vi "StagingBeamLine.vi"() -> ()   [LabVIEW 2020]
uses:
  SubVis/plungerstatus.ctl
  Controls/eventtypdef1.ctl
  Shared/GUI_Template/GUI_master/tcp new data cluster.ctl
panel:
  out "GUIdevice 13":string="StagingImageLocation"
  in  "DigitalOutput.Channel 0::12":bool caption="light"
  out "GUIdevice 12":string="StagingImageLocation"
  in  "JetStages>>JetStages":bool caption="JetStages"
  in  "laser trg":bool caption="Laser Trig."
  in  "Trigger Mode":bool caption="Laser Control"
  in  "Jet>>Jet2":bool caption="JetControl"
  out "ACave Diode Mirror>>XHair":u16(ring) caption="Diode Mirror"
  out "element":T1=enum."IN Beam"
  in  "Position.Channel 6::1":T2(ring) caption="Diode"
  in  "Filpper.Channel 7.Name::1":string="Beam2 Near" caption="Filpper.Channel 5.Name::1"
  in  "Filpper.Channel 6.Name::1":string="Beam2 Near" caption="Filpper.Channel 5.Name::1"
  in  "Position.Channel 7::1":T2(ring) caption="Beam 1 Dump"
  out "Boolean":bool
  in  "Fire button 2":bool caption="OK Button"
  in  "Fire button":bool caption="OK Button"
  in  "Spectrometer>>Spec":bool caption="Spectrometer"
  out "Diode\nFlipper":T3(ring)
  out "Energy\nFilter":T3(ring)
  in  "Uniblitz\nShutter":enum16{"Open", "Close", "Trigger", "Reset"}(ring)=enum."Close"
  out "Phosphor>>Plunger":u16(ring)
  in  "Dutch>>Magnet":bool caption="Mirror"
  out "Wedge>>Plunger":u16(ring)
  out "Beam Dump 2>>Plunger":u16(ring)
  out "Beam Dump 1>>Plunger":u16(ring)
  out "Beam2 Near_1>>XHair":u16(ring)
  out "Beam1 Far_1>>XHair":u16(ring)
  out "Beam1 Near_1>>XHair":u16(ring)
  out "Beam2 Far_2>>XHair":u16(ring)
  out "XH1_3>>XHair":u16(ring)
  in  "position.axis 2::11":dbl=3.999966 caption="OAPstage" min=0.0 max=50.0
  in  "position.axis 3::11":dbl=3.999966 caption="M5stage" min=0.0 max=50.0
  out "GUIdevice 11":string="StagingImageLocation"
  in  "position.channel 2::10":dbl=3.999966 caption="M4stage" min=0.0 max=25.0
  out "GUIdevice 10":string="StagingImageLocation"
  in  "position.channel 1::10":dbl=3.999966 caption="OAPstage" min=0.0 max=25.0
  in  "Position.Axis 5::9":dbl=-19.5 caption="CompPos" min=-49.0 max=51.0
  out "GUIdevice 9":string="StagingTRA3"
  in  "Position.Axis 1::8":dbl=36.99 caption="TelePos" min=0.0 max=150.0
  out "GUIdevice 8":string="StagingTelescopePosition"
  in  "Energy>>Energy":bool
  in  "StagingPhosphor>>Camera":bool caption="Phosphor"
  in  "StagingAlignBeam1>>Camera":bool caption="AlignBeam1"
  in  "StagingAlignBeam2>>Camera":bool caption="AlignBeam2"
  in  "time::7":dbl=-4.151986 caption="time (fs)" min=-2000000.0 max=2000000.0
  out "GUIdevice 7":string="StagingDelayStage"
  in  "position.Axis 1::13":dbl=34.3643 caption="DelayStagePos(mm)" min=0.0 max=54.0
  in  "DeviceControl":bool=TRUE
  in  "ignore interlock::6":bool=TRUE caption="ignore interlock"
  out "GUIdevice 6":string="StagingInterlock"
  out "fire interlock::6":bool caption="Interlock"
  in  "trigger.message::6":string
  in  "enableLaser::5":bool caption="Laser Trig."
  out "GUIdevice 5":string="StagingShotControl"
  out "fire::5":string
  in  "fire!!!":bool caption="fire"
  in  "Mode::5":bool caption="Laser Control"
  in  "position::4":dbl=-39.01 caption="ImagingPos" min=-75.0 max=50.0
  out "GUIdevice 4":string="StagingImageLocation"
  in  "position::3":dbl=10.000035 caption="FocusPos" min=-25.0 max=25.0
  in  "position::2":dbl=3.999966 caption="FocusPos" min=-100.0 max=100.0
  out "GUIdevice 3":string="StagingFocusPositionBeam2"
  out "GUIdevice 2":string="StagingFocusPositionBeam1"
  out "xnames":string[](array[string])=["XH1", "Beam2 Far", "Beam1 Near", "Beam1 Far", "Beam2 Near"]
  out "XHairs":refnum<vi>[](array[refnum])
  out "device status::1":string="no scan"
  in  "Filpper.Channel 5.Name::1":string="Beam2 Near"
  in  "Position.Channel 5::1":T2(ring)
  in  "Filpper.Channel 1.Name::1":string="XH1"
  in  "Filpper.Channel 2.Name::1":string="Beam2 Far"
  in  "Filpper.Channel 3.Name::1":string="Beam1 Near"
  in  "Filpper.Channel 4.Name::1":string="Beam1 Far"
  in  "Position.Channel 1::1":T2(ring)=enum."Unknown"
  in  "Position.Channel 2::1":T2(ring)
  in  "Position.Channel 3::1":T2(ring)
  in  "Position.Channel 4::1":T2(ring)
  out "GUIdevice 1":string="Staging1Wire"
  out "UDP error message":string
  in  "StagingOAP2Far>>Camera":bool caption="OAP2Far"
  in  "StagingOAP2Near>>Camera":bool caption="OAP2Near"
  in  "StagingM5>>Camera":bool caption="M5"
  in  "StagingM1Near>>Camera":bool caption="M1Near"
  in  "StagingM1Far>>Camera":bool caption="M1Far"
  in  "StagingM3Far>>Camera":bool caption="M3"
  in  "StagingM4>>Camera":bool caption="M4"
  in  "StagingOAP1Near>>Camera":bool caption="OAP1Near"
  in  "StagingOAP1Far>>Camera":bool caption="OAP1Far"
  in  "StagingModeTemp>>Camera":bool caption="Mode\nImager"
  in  "Caps>>Caps":bool caption="Caps"
  in  "hexapod>>hexapod":bool caption="hexapod"
  in  "OAP2>>Mirror":bool caption="Mirror"
  in  "DelayStageMotor 2":bool caption="OK Button"
  in  "DelayStageMotor 3":bool caption="OK Button"
  in  "M5>>Mirror":bool caption="Mirror"
  in  "StagingModeImager2>>Camera":bool caption="ModeImager2"
  in  "stop":bool
  in  "M4>>Mirror":bool caption="Mirror"
  in  "OAP1>>Mirror":bool caption="Mirror"
  in  "DelayStageMotor":bool caption="OK Button"
  in  "BS>>Mirror":bool caption="Mirror"
  in  "M1>>Mirror":bool caption="Mirror"
  in  "M3>>Mirror":bool caption="Mirror"
  out "Beam2":bool
  out "Tele":bool
  out "Beam1":bool
  out "after Phos":bool
  out "after Wedge":bool
  out "eBeam":bool
  out "fire":bool=TRUE
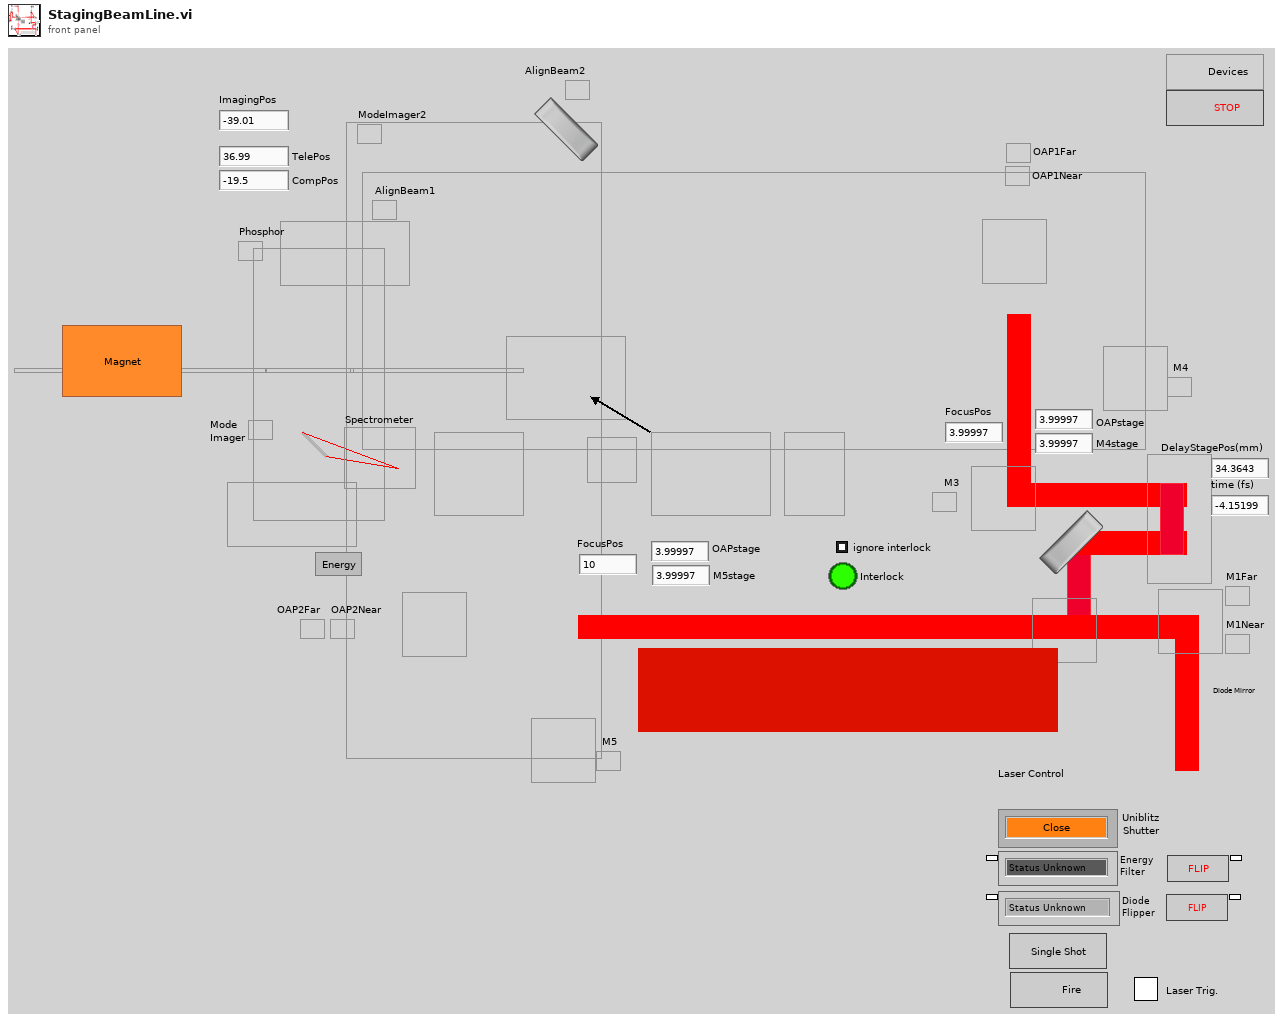
[diagram p1: front panel]
types:
  T1 = typedef "plungerstatus.ctl" = enum16{"unknown", "OUT of Beam", "IN Beam"}
  T2 = enum16{"Removed", "Inserted", "Unknown", "Moving"}
  T3 = enum16{"Status Unknown", "Flipper IN", "Flipper OUT"}
  T4 = enum16{"Read", "Write", "ReadWrite", "BufferedRead", "BufferedReadWrite"}
  T5 = typedef "tcp new data cluster.ctl" = cluster{"EventEnum":enum16{"new data", "connection status update"}, "Device name":string}
  T6 = typedef "eventtypdef1.ctl" = cluster{"label":string, "Sub Panel":refnum<vi>, "CtlRef":refnum<vi>, "This VI":refnum<vi>}
  T7 = enum8{"Enabled", "Disabled", "Disabled and Grayed Out"}
  T8 = enum16{"Beam Dump 1", "Beam Dump 2", "Wedge", "Phosphor"}
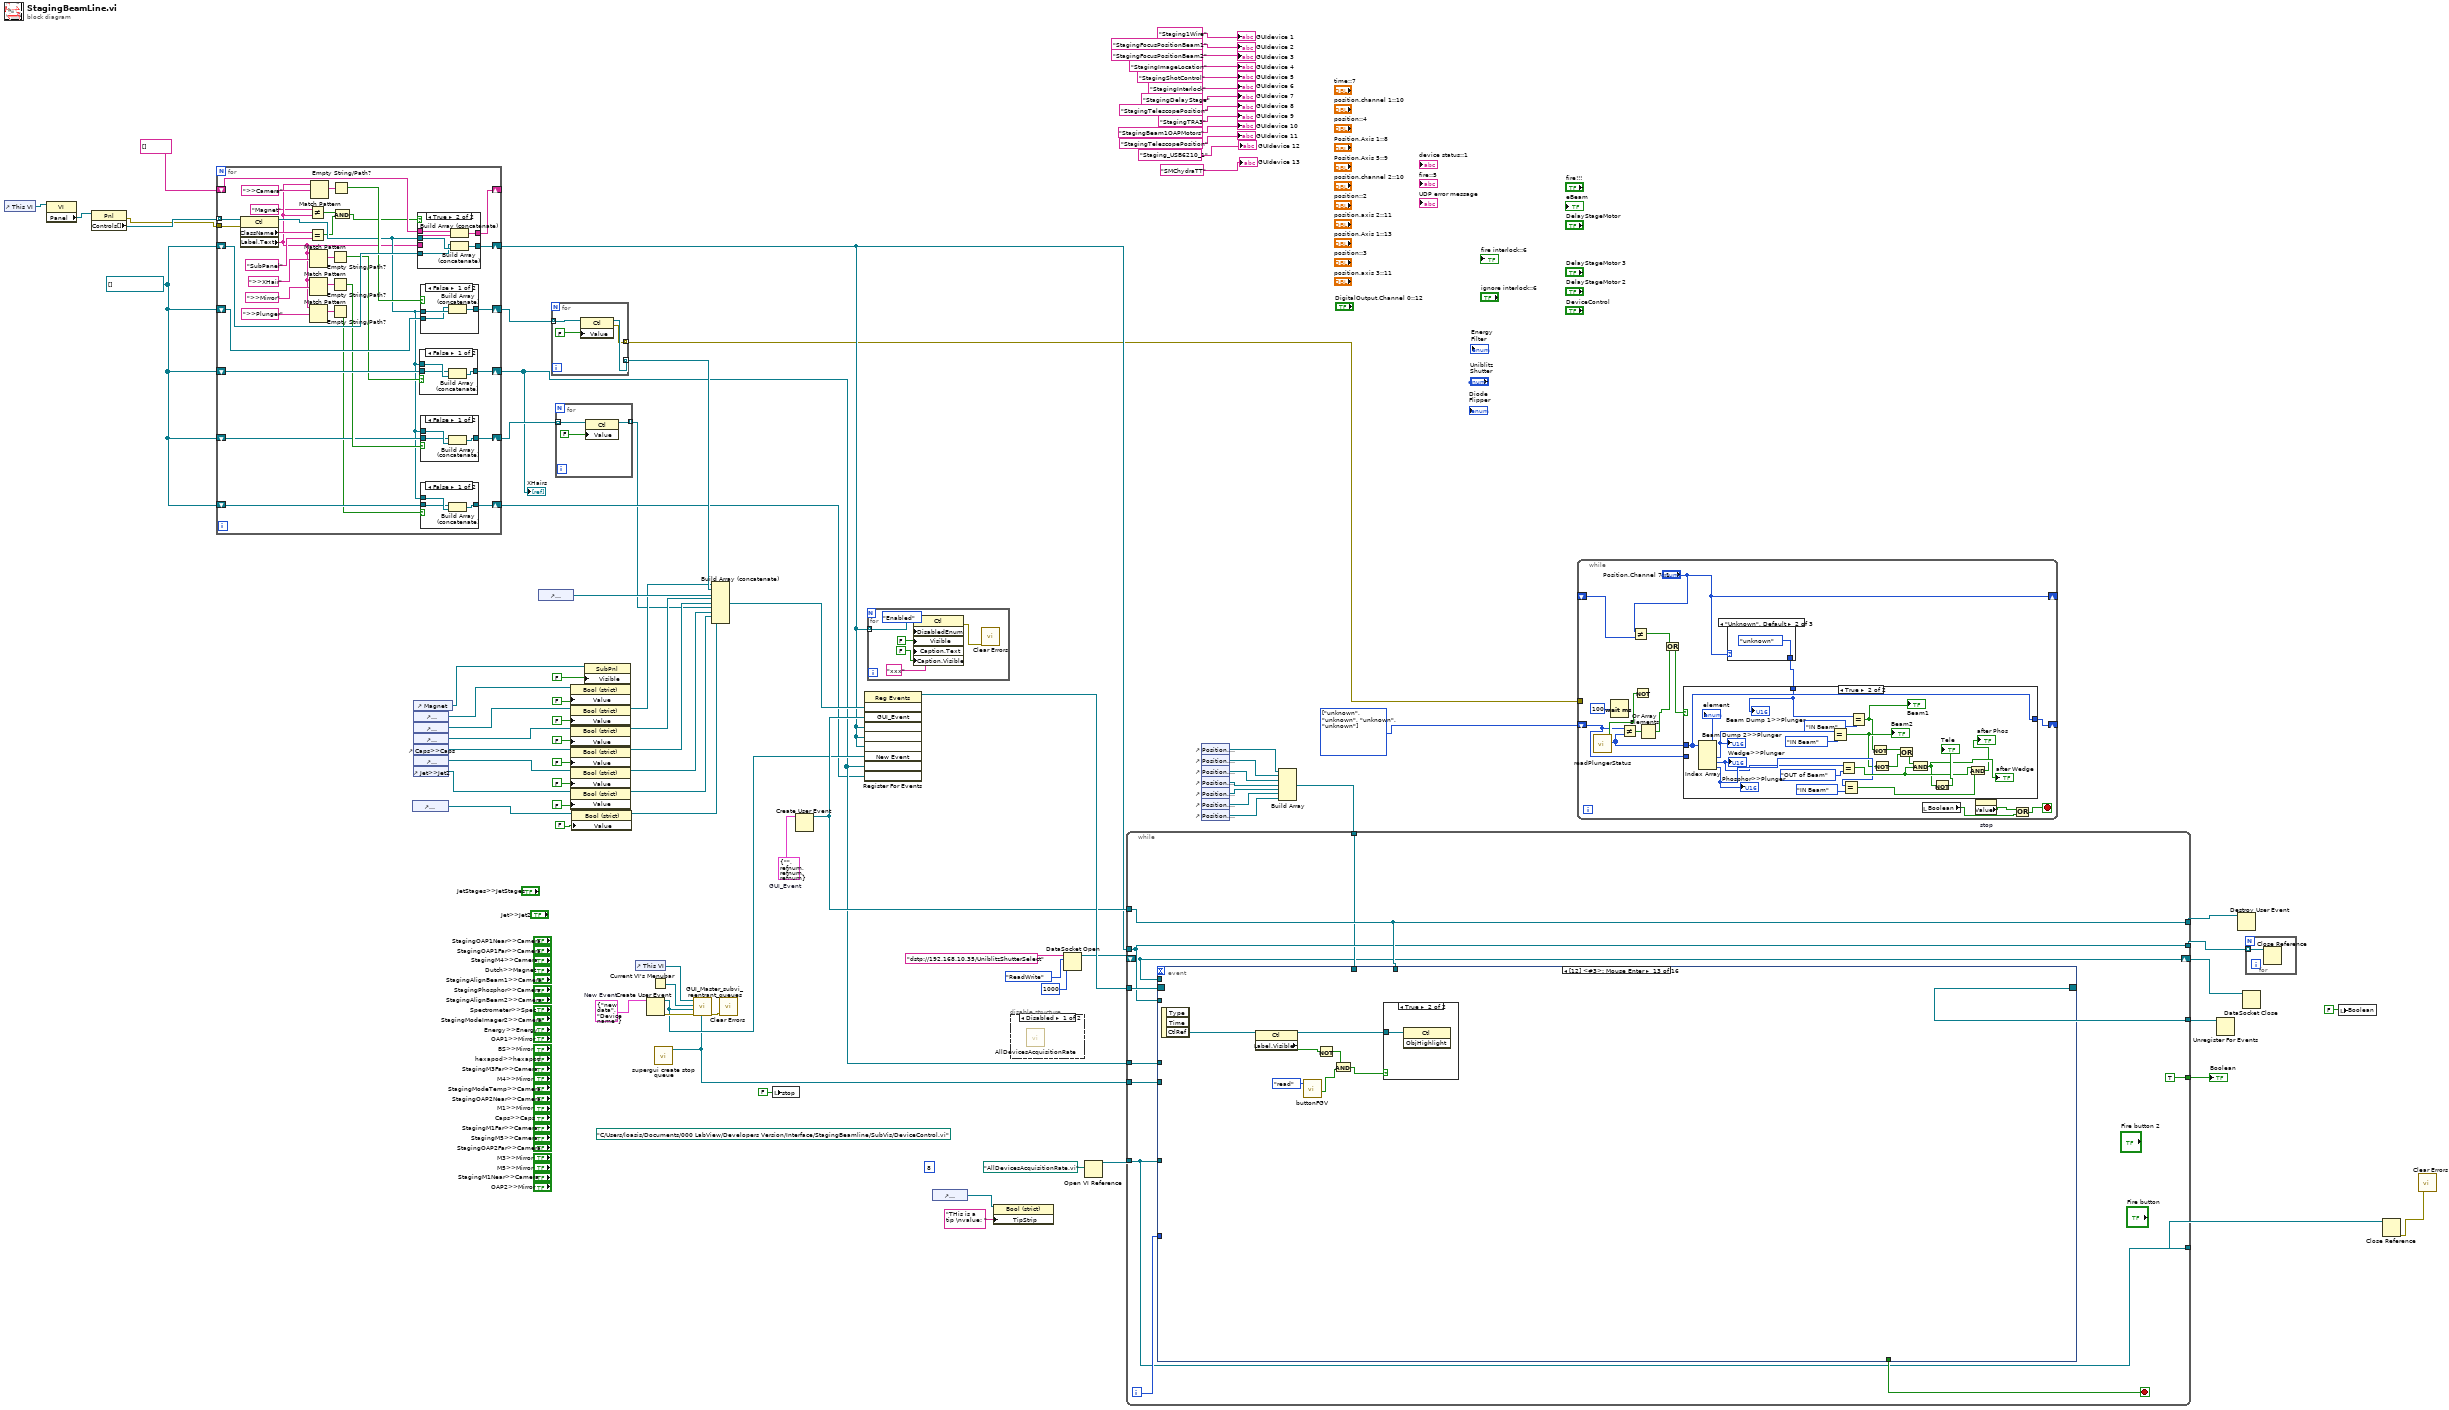
[diagram p0: block diagram]
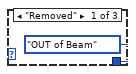
[diagram p2: hidden frame]
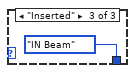
[diagram p3: hidden frame]
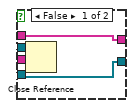
[diagram p10: hidden frame]
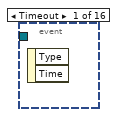
[diagram p11: hidden frame]
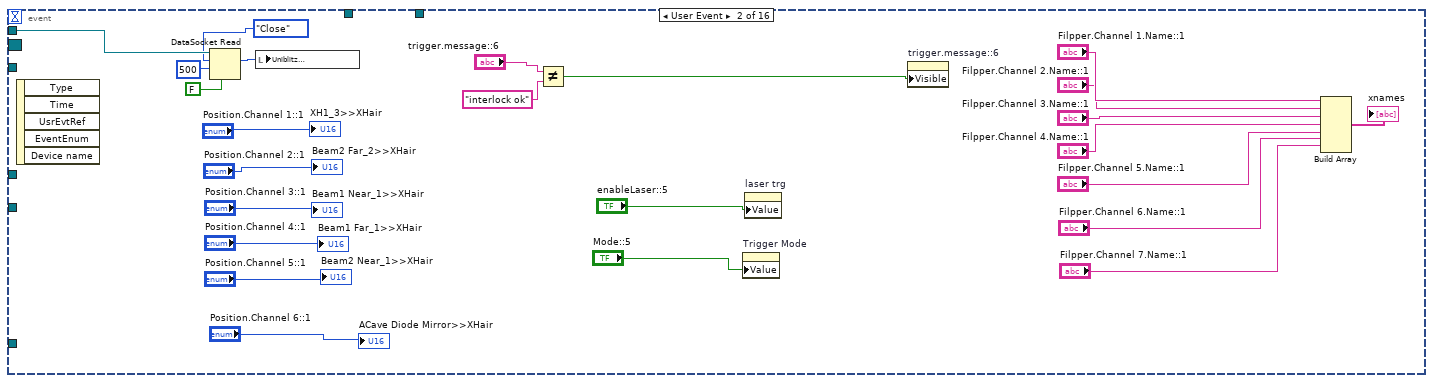
[diagram p12: hidden frame]
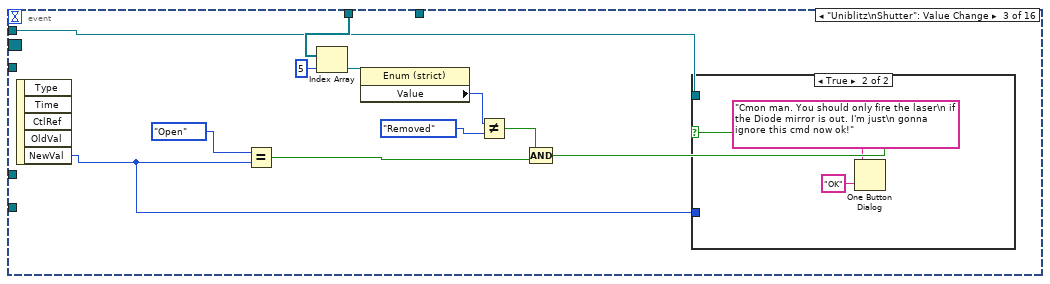
[diagram p13: hidden frame]
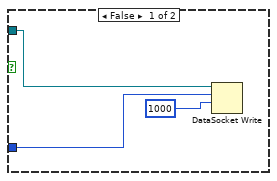
[diagram p14: hidden frame]
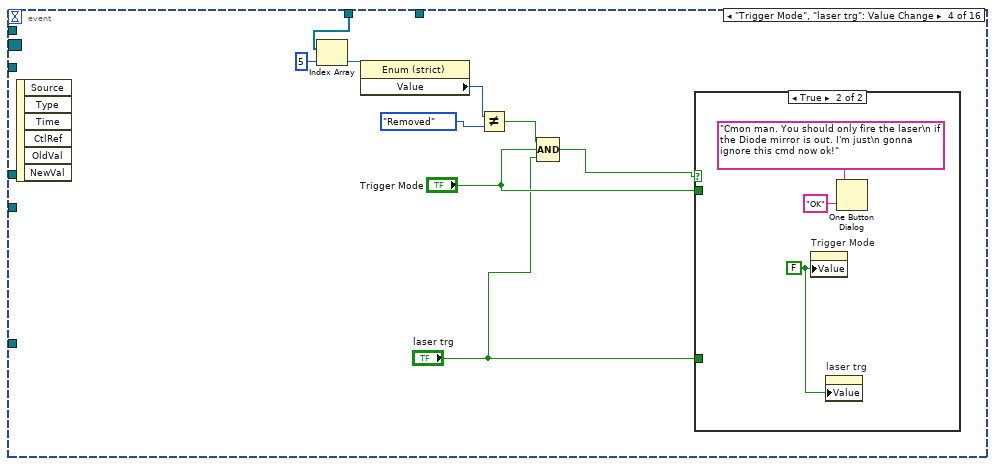
[diagram p15: hidden frame]
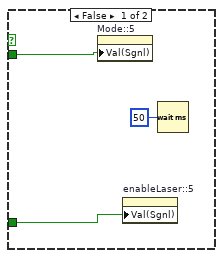
[diagram p16: hidden frame]
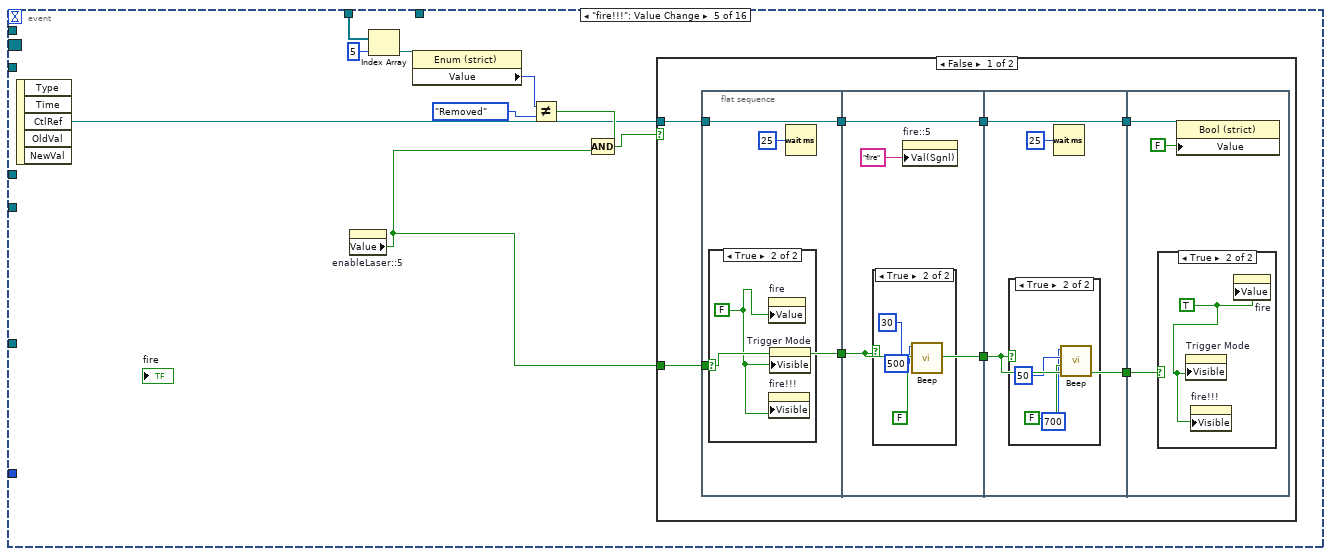
[diagram p17: hidden frame]
diagram:
  w31 = T1[] [enum."unknown", enum."unknown", enum."unknown", enum."unknown"] items=["unknown", "OUT of Beam", "IN Beam"] ("read switches")
  (unwired) path "C:/Users/loasis/Documents/000 LabView/Developers Version/Interface/StagingBeamline/SubVis/DeviceControl.vi" ("Path")
  (unwired) 8 ("options")
  w72 = T5 {"EventEnum"=enum."new data", "Device name"="Device name"}  # New Event
  w40 = refnum<vi>[] []
  w86 = T6 {"label"="", "Sub Panel"=refnum, "CtlRef"=refnum, "This VI"=refnum}  # GUI_Event
  n1 = control-ref of="This VI"() -> (w82:refnum<vi>)
  n2 = property class="VI"(reference=w82) -> ("Panel"=w81:refnum<vi>)  [unwired: 1 in, 2 out]
  n3 = property class="Pnl"(reference=w81) -> (error out=w79:errorcluster, "Controls[]"=w80:refnum<vi>[])  [unwired: 1 in, 1 out]
  n4 = for {
    tunnel: w80 -> [w120] mode=indexing
    tunnel: w79 -> [w121]
    shift-right: [w117] -> _
    shift-left: string[] [] -> [w116]
    shift-right: [w115] -> w75
    shift-left: w40 -> [w114]
    shift-right: [w110] -> w63
    shift-left: w40 -> [w109]
    shift-right: [w108] -> w42
    shift-left: w40 -> [w107]
    shift-right: [w100] -> w53
    shift-left: w40 -> [w99]
    shift-right: [w96] -> w39
    shift-left: w40 -> [w97]
    n5 = property class="Ctl"(reference=w120, error in=w121) -> (reference out=w98:refnum<vi>, "ClassName"=w119:string, "Label.Text"=w92:string)  [unwired: 1 out]
    n6 = Not Equal?(x="Magnet", y=w92) -> (x != y?=w90:bool)
    n7 = Equal?(x=w119, y="SubPanel") -> (x = y?=w88:bool)
    n8 = Match Pattern(string=w92, regular expression=">>XHair") -> (match substring=w105:string)  [unwired: 1 in, 3 out]
    n9 = Match Pattern(string=w92, regular expression=">>Mirror") -> (match substring=w102:string)  [unwired: 1 in, 3 out]
    n10 = Match Pattern(string=w92, regular expression=">>Plunger") -> (match substring=w94:string)  [unwired: 1 in, 3 out]
    n11 = Match Pattern(string=w92, regular expression=">>Camera") -> (match substring=w112:string)  [unwired: 1 in, 3 out]
    n12 = Empty String/Path?(string/path=w105) -> (empty?=w104:bool)
    n13 = Empty String/Path?(string/path=w102) -> (empty?=w103:bool)
    n14 = Empty String/Path?(string/path=w94) -> (empty?=w93:bool)
    n15 = Empty String/Path?(string/path=w112) -> (empty?=w111:bool)
    n16 = And(x=w90, y=w88) -> (x .and. y?=w89:bool)
    n17 = case shown="True" w89 {
      tunnel: w98 -> [w140 w143]
      tunnel: w92 -> [_ w146]
      tunnel: [w139 w145] -> w117
      tunnel: w116 -> [w139 w144]
      tunnel: [w138 w142] -> w115
      tunnel: w114 -> [w138 w141]
      frame False {
        n18 = Close Reference(reference=w140) -> ()  [unwired: 1 in, 1 out]
      }
      frame True {
        n19 = Build Array (concatenate)(w144, w146) -> (w145:string[])
        n20 = Build Array (concatenate)(w141, w143) -> (w142:refnum<vi>[])
      }
    }
    n21 = case shown="False" w104 {
      tunnel: w98 -> [w132 _]
      tunnel: [w131 w133] -> w108
      tunnel: w107 -> [w130 w133]
      frame False {
        n22 = Build Array (concatenate)(w130, w132) -> (w131:refnum<vi>[])
      }
      frame True {
      }
    }
    n23 = case shown="False" w111 {
      tunnel: w98 -> [w136 _]
      tunnel: [w135 w137] -> w110
      tunnel: w109 -> [w134 w137]
      frame False {
        n24 = Build Array (concatenate)(w134, w136) -> (w135:refnum<vi>[])
      }
      frame True {
      }
    }
    n25 = case shown="False" w103 {
      tunnel: w98 -> [w128 _]
      tunnel: [w127 w129] -> w100
      tunnel: w99 -> [w126 w129]
      frame False {
        n26 = Build Array (concatenate)(w126, w128) -> (w127:refnum<vi>[])
      }
      frame True {
      }
    }
    n27 = case shown="False" w93 {
      tunnel: w98 -> [w124 _]
      tunnel: [w123 w125] -> w96
      tunnel: w97 -> [w122 w125]
      frame False {
        n28 = Build Array (concatenate)(w122, w124) -> (w123:refnum<vi>[])
      }
      frame True {
      }
    }
  }
  "XHairs" <- w42
  n29 = control-ref of="JetStages>>JetStages"() -> (w5:refnum<vi>)
  n30 = control-ref of="Magnet"() -> (w35:refnum<vi>)
  n31 = control-ref of="Dutch>>Magnet"() -> (w38:refnum<vi>)
  n32 = control-ref of="Energy>>Energy"() -> (w49:refnum<vi>)
  n33 = control-ref of="hexapod>>hexapod"() -> (w59:refnum<vi>)
  n34 = control-ref of="Caps>>Caps"() -> (w61:refnum<vi>)
  n35 = control-ref of="Spectrometer>>Spec"() -> (w34:refnum<vi>)
  n36 = control-ref of="Jet>>Jet2"() -> (w16:refnum<vi>)
  n37 = control-ref of="StagingModeImager2>>Camera"() -> (w85:refnum<vi>)
  n38 = for {
    tunnel: w63 -> [w150] mode=indexing
    tunnel: [w148] -> w62 mode=indexing
    tunnel: [w147] -> w27 mode=indexing
    n39 = property class="Ctl"(reference=w150, "Value"=FALSE ("Visible")) -> (reference out=w148:refnum<vi>, error out=w147:errorcluster)  [unwired: 1 in]
  }
  n40 = for {
    tunnel: w53 -> [w153] mode=indexing
    tunnel: [w151] -> w14 mode=indexing
    n41 = property class="Ctl"(reference=w153, "Value"=FALSE ("Visible")) -> (reference out=w151:refnum<vi>)  [unwired: 1 in, 1 out]
  }
  n42 = property class="Bool (strict)"(reference=w38, "Value"=FALSE) -> ()  [unwired: 1 in, 2 out]
  n43 = property class="Bool (strict)"(reference=w49, "Value"=FALSE) -> (reference out=w47:refnum<vi>)  [unwired: 1 in, 1 out]
  n44 = property class="Bool (strict)"(reference=w59, "Value"=FALSE) -> (reference out=w58:refnum<vi>)  [unwired: 1 in, 1 out]
  n45 = property class="Bool (strict)"(reference=w61, "Value"=FALSE) -> (reference out=w19:refnum<vi>)  [unwired: 1 in, 1 out]
  n46 = property class="Bool (strict)"(reference=w34, "Value"=FALSE) -> (reference out=w32:refnum<vi>)  [unwired: 1 in, 1 out]
  n47 = property class="Bool (strict)"(reference=w16, "Value"=FALSE) -> (reference out=w15:refnum<vi>)  [unwired: 1 in, 1 out]
  n48 = property class="Bool (strict)"(reference=w5, "Value"=FALSE) -> (reference out=w4:refnum<vi>)  [unwired: 1 in, 1 out]
  n49 = property class="SubPnl"(reference=w35, "Visible"=FALSE) -> ()  [unwired: 1 in, 2 out]
  n50 = control-ref of="This VI"() -> (w70:refnum<vi>)
  n51 = Create User Event(user event datatype=w72) -> (user event=w69:refnum<user-event>, error out=w73:errorcluster)  [unwired: 1 in]
  n52 = Current VI's Menubar() -> (w71:refnum<k9>)
  n53 = call "supergui create stop queue.vi"() -> ("STOP Queue out"=w1:refnum<queue>)  [unwired: 11 in]
  n54 = call "GUI_Master_subvi_reentrant_queues.vi"("STOP Queue in"=w1, "error in (no error)"=w73, "tcp data event"=w69, "Caller menu reference"=w71, "Caller VI ref"=w70) -> ("error out"=w74:errorcluster)  [unwired: 6 in]
  n55 = Build Array (concatenate)(w47, w62, w85, w58, w19, w14, w32, w15, w4) -> (w84:refnum<vi>[])
  n56 = call <vilib>:"Clear Errors.vi"("error in (no error)"=w74) -> ()  [unwired: 5 in, 2 out]
  n57 = local write "stop"(FALSE ("stop")) -> ()
  n58 = Create User Event(user event datatype=w86) -> (user event=w76:refnum<user-event>)  [unwired: 1 in, 1 out]
  n59 = register-events(w84, w76, w75, w75, w75, w69, w42, w39) -> (reference out=w83:refnum<event-registration>)  [unwired: 2 in, 1 out]
  n60 = for {
    tunnel: w75 -> [w158] mode=indexing
    n61 = property class="Ctl"(reference=w158, "DisabledEnum"=T7."Enabled" ("Disabled"), "Visible"=FALSE, "Caption.Text"="xxx", "Caption.Visible"=FALSE ("Label.Visible")) -> (error out=w154:errorcluster)  [unwired: 1 in, 1 out]
    n62 = call <vilib>:"Clear Errors.vi"("error in (no error)"=w154) -> ()  [unwired: 5 in, 2 out]
  }
  n63 = control-ref of="DelayStageMotor"() -> (w44:refnum<vi>)
  n64 = property class="Bool (strict)"(reference=w44, "TipStrip"="THis is a tip \nvalue: ") -> ()  [unwired: 1 in, 2 out]
  n65 = disable-structure shown="Disabled" {
    frame Disabled {
      n66 = call "AllDevicesAcquisitionRate.vi"() -> ()  [unwired: 11 in, 1 out]
    }
    frame Enabled {
    }
  }
  n67 = DataSocket Open(9:1000 ("ms timeout (10000)"), 10:T4."ReadWrite" ("mode"), 11:"dstp://192.168.10.35/UniblitzShutterSelect" ("URL")) -> (3:w26:refnum<k13>)  [unwired: 1 in, 1 out]
  n68 = Open VI Reference(vi path=path "AllDevicesAcquisitionRate.vi" ("Path")) -> (vi reference=w54:refnum<vi>)  [unwired: 5 in, 1 out]
  n69 = control-ref of="Position.Channel 1::1"() -> (w64:refnum<vi>)
  n70 = control-ref of="Position.Channel 2::1"() -> (w65:refnum<vi>)
  n71 = control-ref of="Position.Channel 3::1"() -> (w66:refnum<vi>)
  n72 = control-ref of="Position.Channel 4::1"() -> (w67:refnum<vi>)
  n73 = control-ref of="Position.Channel 5::1"() -> (w68:refnum<vi>)
  n74 = control-ref of="Position.Channel 6::1"() -> (w21:refnum<vi>)
  n75 = control-ref of="Position.Channel 7::1"() -> (w20:refnum<vi>)
  n76 = Build Array(w64, w65, w66, w67, w68, w21, w20) -> (w18:refnum<vi>[])
  n77 = while {
    tunnel: w76 -> [w170]
    tunnel: [w170] -> w87
    tunnel: w83 -> [w169]
    tunnel: w75 -> [w168]
    tunnel: [w168] -> w77
    tunnel: w42 -> [w166]
    tunnel: w18 -> [w165]
    tunnel: [w164] -> w56
    tunnel: w54 -> [w164]
    tunnel: [w163] -> w41
    tunnel: [TRUE] -> w29
    shift-right: [w161] -> w25
    shift-left: w26 -> [w161]
    tunnel: w1 -> [w160]
    i -> [w167]
    stop <- w171 stop-if-true
    n78 = event shown="[12] <#3>: Mouse Enter" {
      selector: w169 -> [_ _ _ _ _ _ _ _ _ _ _ _ _ _ _ _]
      dyn-events: [_ _ _ _ _ _ _ _ _ _ _ _ _ _ _ _] -> w163
      timeout: _ -> [_ _ _ _ _ _ _ _ _ _ _ _ _ _ _ _]
      tunnel: [_ _ _ _ _ _ _ _ _ _ _ _ _ _ _ "stop"] -> w171
      tunnel: w170 -> [_ _ _ _ _ _ _ _ w305 w309 _ _ _ _ _ w395]
      tunnel: w168 -> [_ _ _ _ _ _ _ _ w304 w307 _ w334 _ _ _ _]
      tunnel: w167 -> [_ _ _ _ _ _ _ _ _ _ _ _ _ _ _ _]
      tunnel: w166 -> [_ _ _ _ _ _ _ _ _ _ _ _ _ _ _ _]
      tunnel: w165 -> [_ _ w206 w216 w231 w276 _ _ _ _ _ _ _ _ _ _]
      tunnel: w164 -> [_ _ _ _ _ _ _ _ _ _ w317 _ _ _ _ _]
      tunnel: w161 -> [_ w181 w196 _ _ _ _ _ _ _ _ _ _ _ _ _]
      tunnel: w160 -> [_ _ _ _ _ _ _ _ _ _ _ _ _ _ _ w388]
      event Timeout {
        n79 = event-data() -> ()  [unwired: 1 in, 2 out]
      }
      event User Event {
        n80 = event-data() -> ()  [unwired: 1 in, 5 out]
        n81 = DataSocket Read(6:FALSE ("wait for updated value (T)"), 9:500 ("ms timeout (10000)"), 10:enum16{"Open", "Close", "Trigger", "Reset"}."Close" ("Uniblitz\nShutter 2"), 11:w181) -> (2:w179:enum16{"Open", "Close", "Trigger", "Reset"})  [unwired: 1 in, 6 out]
        n82 = local write "Uniblitz\nShutter"(w179) -> ()
        n83 = Not Equal?(x="trigger.message::6", y="interlock ok") -> (x != y?=w182:bool)
        n84 = property on="Trigger Mode" class="Bool (strict)"("Value"="Mode::5") -> ()  [unwired: 2 in, 2 out]
        n85 = property on="laser trg" class="Bool (strict)"("Value"="enableLaser::5") -> ()  [unwired: 2 in, 2 out]
        n86 = property on="trigger.message::6" class="Str"("Visible"=w182) -> ()  [unwired: 2 in, 2 out]
        n87 = Build Array("Filpper.Channel 1.Name::1", "Filpper.Channel 2.Name::1", "Filpper.Channel 3.Name::1", "Filpper.Channel 4.Name::1", "Filpper.Channel 5.Name::1", "Filpper.Channel 6.Name::1", "Filpper.Channel 7.Name::1") -> (→"xnames":string[])
        "XH1_3>>XHair" <- "Position.Channel 1::1"
        "Beam2 Far_2>>XHair" <- "Position.Channel 2::1"
        "Beam1 Near_1>>XHair" <- "Position.Channel 3::1"
        "Beam1 Far_1>>XHair" <- "Position.Channel 4::1"
        "Beam2 Near_1>>XHair" <- "Position.Channel 5::1"
        "ACave Diode Mirror>>XHair" <- "Position.Channel 6::1"
      }
      event "Uniblitz\nShutter": Value Change {
        n88 = event-data() -> ("NewVal"=w197:enum16{"Open", "Close", "Trigger", "Reset"})  [unwired: 1 in, 4 out]
        n89 = Equal?(x=enum16{"Open", "Close", "Trigger", "Reset"}."Open" ("Uniblitz\nShutter"), y=w197) -> (x = y?=w199:bool)
        n90 = Index Array(array=w206, index=5) -> (element=w204:refnum<vi>)
        n91 = property class="Enum (strict)"(reference=w204) -> ("Value"=w201:T2)  [unwired: 1 in, 2 out]
        n92 = Not Equal?(x=w201, y=T2."Removed" ("Position.Channel 6::1")) -> (x != y?=w200:bool)
        n93 = Compound Arithmetic op=AND(w200, w199) -> (w198:bool)
        n94 = case shown="True" w198 {
          tunnel: w197 -> [w208 _]
          tunnel: w196 -> [w207 _]
          frame False {
            n95 = DataSocket Write(9:1000 ("ms timeout (0)"), 10:w208, 11:w207) -> ()  [unwired: 1 in, 3 out]
          }
          frame True {
            n96 = One Button Dialog(message="Cmon man. You should only fire the laser\n if the Diode mirror is out. I'm just\n gonna ignore this cmd now ok!", button name ("OK")="OK") -> ()  [unwired: 1 out]
          }
        }
      }
      event "Trigger Mode", "laser trg": Value Change {
        n97 = event-data() -> ()  [unwired: 1 in, 6 out]
        n98 = Index Array(array=w216, index=5) -> (element=w219:refnum<vi>)
        n99 = property class="Enum (strict)"(reference=w219) -> ("Value"=w217:T2)  [unwired: 1 in, 2 out]
        n100 = Not Equal?(x=w217, y=T2."Removed" ("Position.Channel 6::1")) -> (x != y?=w215:bool)
        n101 = Compound Arithmetic op=AND(w215, "Trigger Mode", "laser trg") -> (w214:bool)
        n102 = case shown="True" w214 {
          tunnel: "Trigger Mode" -> [w223 _]
          tunnel: "laser trg" -> [w222 _]
          frame False {
            n103 = property on="Mode::5" class="Bool (strict)"("Val(Sgnl)"=w223) -> ()  [unwired: 2 in, 2 out]
            n104 = property on="enableLaser::5" class="Bool (strict)"("Val(Sgnl)"=w222) -> ()  [unwired: 2 in, 2 out]
            n105 = Wait (ms)(milliseconds to wait=u32 50) -> ()  [unwired: 1 out]
          }
          frame True {
            w224 = FALSE ("Trigger Mode")
            n106 = property on="Trigger Mode" class="Bool (strict)"("Value"=w224) -> ()  [unwired: 2 in, 2 out]
            n107 = property on="laser trg" class="Bool (strict)"("Value"=w224) -> ()  [unwired: 2 in, 2 out]
            n108 = One Button Dialog(message="Cmon man. You should only fire the laser\n if the Diode mirror is out. I'm just\n gonna ignore this cmd now ok!", button name ("OK")="OK") -> ()  [unwired: 1 out]
          }
        }
      }
      event "fire!!!": Value Change {
        n109 = event-data() -> ("CtlRef"=w228:refnum<vi>)  [unwired: 1 in, 4 out]
        n110 = property on="enableLaser::5" class="Bool (strict)"() -> ("Value"=w227:bool)  [unwired: 2 in, 2 out]
        n111 = Index Array(array=w231, index=5) -> (element=w234:refnum<vi>)
        n112 = property class="Enum (strict)"(reference=w234) -> ("Value"=w232:T2)  [unwired: 1 in, 2 out]
        n113 = Not Equal?(x=w232, y=T2."Removed" ("Position.Channel 6::1")) -> (x != y?=w230:bool)
        n114 = Compound Arithmetic op=AND(w230, w227) -> (w229:bool)
        n115 = case shown="False" w229 {
          tunnel: w228 -> [w240 w264]
          tunnel: w227 -> [w239 _]
          frame False {
            n116 = flat-sequence {
              tunnel: [w245] -> w241
              tunnel: w240 -> [w245]
              tunnel: w239 -> [w244]
              tunnel: [w244] -> w238
              tunnel: [w249] -> w242
              tunnel: w241 -> [w249]
              tunnel: w238 -> [w248]
              tunnel: [w248] -> w237
              tunnel: [w255] -> w243
              tunnel: w242 -> [w255]
              tunnel: w237 -> [w254]
              tunnel: [w254] -> w236
              tunnel: w243 -> [w261]
              tunnel: w236 -> [w260]
              frame #0 {
                n117 = case shown="True" w244 {
                  frame False {
                  }
                  frame True {
                    w247 = FALSE ("fire ind")
                    n118 = property on="fire" class="Bool (strict)"("Value"=w247) -> ()  [unwired: 2 in, 2 out]
                    n119 = property on="fire!!!" class="Bool (strict)"("Visible"=w247) -> ()  [unwired: 2 in, 2 out]
                    n120 = property on="Trigger Mode" class="Bool (strict)"("Visible"=w247) -> ()  [unwired: 2 in, 2 out]
                  }
                }
                n121 = Wait (ms)(milliseconds to wait=u32 25) -> ()  [unwired: 1 out]
              }
              frame #1 {
                n122 = case shown="True" w248 {
                  frame False {
                  }
                  frame True {
                    n123 = call <vilib>:"Beep.vi"("use system alert? (T)"=FALSE ("use system alert? (T) 2"), "duration (msec)"=u32 30 ("duration (msec) 2"), "frequency (Hz)"=u32 500 ("frequency (Hz) 2")) -> ()  [unwired: 9 in]
                  }
                }
                n124 = property on="fire::5" class="Str"("Val(Sgnl)"="fire" ("fire::5")) -> ()  [unwired: 2 in, 2 out]
              }
              frame #2 {
                n125 = case shown="True" w254 {
                  frame False {
                  }
                  frame True {
                    n126 = call <vilib>:"Beep.vi"("use system alert? (T)"=FALSE, "duration (msec)"=u32 50, "frequency (Hz)"=u32 700) -> ()  [unwired: 9 in]
                  }
                }
                n127 = Wait (ms)(milliseconds to wait=u32 25) -> ()  [unwired: 1 out]
              }
              frame #3 {
                n128 = case shown="True" w260 {
                  frame False {
                  }
                  frame True {
                    w263 = TRUE ("fire ind")
                    n129 = property on="Trigger Mode" class="Bool (strict)"("Visible"=w263) -> ()  [unwired: 2 in, 2 out]
                    n130 = property on="fire!!!" class="Bool (strict)"("Visible"=w263) -> ()  [unwired: 2 in, 2 out]
                    n131 = property on="fire" class="Bool (strict)"("Value"=w263) -> ()  [unwired: 2 in, 2 out]
                  }
                }
                n132 = property class="Bool (strict)"(reference=w261, "Value"=FALSE) -> ()  [unwired: 1 in, 2 out]
              }
            }
          }
          frame True {
            n133 = One Button Dialog(message="Cmon man. You should only fire the laser\n if the Diode mirror is out. I'm just\n gonna ignore this cmd now ok!", button name ("OK")="OK") -> ()  [unwired: 1 out]
            n134 = property class="Bool (strict)"(reference=w264, "Value"=FALSE) -> ()  [unwired: 1 in, 2 out]
          }
        }
      }
      event Mouse Down {
        w270 = T2."Removed" ("y")
        n135 = event-data() -> ("CtlRef"=w278:refnum<vi>)  [unwired: 1 in, 6 out]
        n136 = property class="Ctl"(reference=w278) -> ("Label.Text"=w283:string)  [unwired: 1 in, 2 out]
        n137 = Match Pattern(string=w283, regular expression=">>") -> (before substring=w281:string)  [unwired: 1 in, 3 out]
        n138 = local read "xnames"() -> (w277:string[])
        n139 = Match Pattern(string=w281, regular expression="_") -> (before substring=w279:string)  [unwired: 1 in, 3 out]
        n140 = Search 1D Array(1D array=w277, element=w279) -> (index of element=w275:i32)  [unwired: 1 in]
        n141 = Index Array(array=w276, index=w275) -> (element=w274:refnum<vi>)
        n142 = property class="Enum (strict)"(reference=w274) -> (reference out=w269:refnum<vi>, "Value"=w273:T2)  [unwired: 1 in, 1 out]
        n143 = Equal?(x=w273, y=w270) -> (x = y?=w272:bool)
        n144 = Select(t=T2."Inserted" ("y"), s=w272, f=w270) -> (s? t:f=w268:T2)
        n145 = property class="Enum (strict)"(reference=w269, "Val(Sgnl)"=w268) -> ()  [unwired: 1 in, 2 out]
      }
      event "Beam Dump 1>>Plunger": Mouse Down {
        w286 = T2."Removed" ("y")
        n146 = event-data() -> ()  [unwired: 1 in, 8 out]
        n147 = property on="Beam Dump 1>>Plunger" class="Ring (strict)"() -> ("Value"=w289:u16)  [unwired: 2 in, 2 out]
        n148 = case shown="0, Default" w289 {
          tunnel: [T2."Unknown" ("Position.Channel 7::1") T2."Removed" ("Position.Channel 7::1") T2."Inserted" ("Position.Channel 7::1")] -> w285
          frame 0, Default {
          }
          frame 1 {
          }
          frame 2 {
          }
        }
        n149 = Equal?(x=w285, y=w286) -> (x = y?=w288:bool)
        n150 = Select(t=T2."Inserted" ("y"), s=w288, f=w286) -> (s? t:f=w284:T2)
        n151 = property on="Position.Channel 7::1" class="Enum (strict)"("Val(Sgnl)"=w284) -> ()  [unwired: 2 in, 2 out]
      }
      event Mouse Down? {
        n152 = event-data() -> ("CtlRef"=w296:refnum<vi>)  [unwired: 1 in, 6 out]
        n153 = property class="Ctl"(reference=w296) -> ("Label.Text"=w300:string)  [unwired: 1 in, 2 out]
        n154 = Match Pattern(string=w300, regular expression=">>") -> (before substring=w298:string)  [unwired: 1 in, 3 out]
        n155 = Match Pattern(string=w298, regular expression="_") -> (before substring=w295:string)  [unwired: 1 in, 3 out]
        n156 = Scan From String(input string=w295, default 1=T8."Phosphor" ("Plunger")) -> (output 1=w293:T8)  [unwired: 3 in, 3 out]
        n157 = disable-structure shown="Enabled" {
          disable-tunnel: w293 -> [w302 _]
          frame Enabled {
            n158 = call "toggle Plunger.vi"("Plunger"=w302) -> ("error out"=w301:errorcluster)  [unwired: 10 in]
            n159 = call <vilib>:"Clear Errors.vi"("error in (no error)"=w301) -> ()  [unwired: 5 in, 2 out]
          }
          frame Disabled {
          }
        }
        n160 = event-data() -> ()  [unwired: 5 in, 1 out]
      }
      event Mouse Down {
        n161 = event-data() -> ("CtlRef"=w303:refnum<vi>)  [unwired: 1 in, 6 out]
        n162 = call "LaunchGUI.vi"("Array"=w304, "CtlRef"=w303, "User Event in"=w305) -> ()  [unwired: 9 in]
      }
      event "Dutch>>Magnet": Value Change {
        n163 = event-data() -> ("CtlRef"=w308:refnum<vi>, "NewVal"=w306:bool)  [unwired: 1 in, 3 out]
        n164 = case shown="True" w306 {
          tunnel: w309 -> [_ w316]
          tunnel: w308 -> [_ w314]
          tunnel: w307 -> [_ w313]
          frame False {
          }
          frame True {
            n165 = control-ref of="Magnet"() -> (w312:refnum<vi>)
            n166 = call "buttonFGV.vi"("command"=enum16{"read", "write"}."write", "Boolean in"=w314) -> ()  [unwired: 7 in, 3 out]
            n167 = property class="SubPnl"(reference=w312, "Visible"=TRUE) -> (reference out=w311:refnum<vi>)  [unwired: 1 in, 1 out]
            n168 = call "LaunchGUI.vi"("Array"=w313, "CtlRef"=w311, "User Event in"=w316) -> ()  [unwired: 9 in]
          }
        }
      }
      event "DeviceControl": Value Change {
        n169 = event-data() -> ("CtlRef"=w319:refnum<vi>, "NewVal"=w318:bool)  [unwired: 1 in, 3 out]
        n170 = case shown="False" w318 {
          tunnel: w317 -> [w326 _]
          tunnel: w319 -> [w320 _]
          frame False {
            n171 = invoke class="VI" method="FP.Open"(reference=w326) -> (reference out=w323:refnum<vi>)  [unwired: 4 in, 4 out]
            n172 = invoke class="VI" method="Ctrl Val.Set"(reference=w323, "Control Name"="stop", "Value"=w320) -> (reference out=w322:refnum<vi>)  [unwired: 2 in, 4 out]
            n173 = invoke class="VI" method="Run VI"(reference=w322, "Wait until done"=FALSE ("Wait Until Done"), "Auto Dispose Ref"=FALSE ("Auto Dispose Reference")) -> ()  [unwired: 2 in, 5 out]
          }
          frame True {
          }
        }
      }
      event Value Change {
        n174 = event-data() -> ("CtlRef"=w329:refnum<vi>, "OldVal"=w332:variant)  [unwired: 1 in, 3 out]
        n175 = Variant To Data(type=FALSE, Variant=w332) -> (data=w330:bool)  [unwired: 1 in, 1 out]
        n176 = To More Specific Class(target class=refnum<vi> refnum ("Boolean in"), reference=w329) -> (specific class reference=w328:refnum<vi>)  [unwired: 1 in, 1 out]
        n177 = property class="Bool (strict)"(reference=w328, "Value"=TRUE) -> ()  [unwired: 1 in, 2 out]
        n178 = case shown="False" w330 {
          tunnel: w334 -> [w338 _]
          tunnel: w328 -> [w335 _]
          frame False {
            n179 = call "buttonFGV.vi"("command"=enum16{"read", "write"}."write", "Boolean in"=w335) -> ()  [unwired: 7 in, 3 out]
            n180 = for {
              tunnel: w338 -> [w340] mode=indexing
              n181 = property class="Ctl"(reference=w340, "Visible"=TRUE) -> ()  [unwired: 1 in, 2 out]
            }
            n182 = property class="Bool (strict)"(reference=w335, "Value"=TRUE) -> (error out=w336:errorcluster)  [unwired: 1 in, 1 out]
            n183 = call <vilib>:"Clear Errors.vi"("error in (no error)"=w336) -> ()  [unwired: 5 in, 2 out]
          }
          frame True {
          }
        }
      }
      event Mouse Enter {
        n184 = event-data() -> ("CtlRef"=w347:refnum<vi>)  [unwired: 1 in, 2 out]
        n185 = property class="Ctl"(reference=w347) -> (reference out=w346:refnum<vi>, "Label.Visible"=w345:bool)  [unwired: 1 in, 1 out]
        n186 = call "buttonFGV.vi"("command"=enum16{"read", "write", "clear"}."read" ("Enum")) -> ("select subPanel"=w343:bool)  [unwired: 8 in, 2 out]
        n187 = Not(x=w345) -> (.not. x?=w344:bool)
        n188 = And(x=w344, y=w343) -> (x .and. y?=w342:bool)
        n189 = case shown="True" w342 {
          tunnel: w346 -> [_ w349]
          frame False {
          }
          frame True {
            n190 = invoke class="Ctl" method="ObjHighlight"(reference=w349) -> ()  [unwired: 2 in, 3 out]
          }
        }
      }
      event Mouse Leave {
        n191 = event-data() -> ("CtlRef"=w356:refnum<vi>)  [unwired: 1 in, 2 out]
        n192 = property class="Ctl"(reference=w356) -> (reference out=w355:refnum<vi>, error out=w350:errorcluster, "Caption.Visible"=w354:bool)  [unwired: 1 in]
        n193 = call "buttonFGV.vi"("command"=enum16{"read", "write", "clear"}."read" ("Enum")) -> ("select subPanel"=w352:bool)  [unwired: 8 in, 2 out]
        n194 = Not(x=w354) -> (.not. x?=w353:bool)
        n195 = And(x=w353, y=w352) -> (x .and. y?=w351:bool)
        n196 = call <vilib>:"Clear Errors.vi"("error in (no error)"=w350) -> ()  [unwired: 5 in, 2 out]
        n197 = case shown="True" w351 {
          tunnel: w355 -> [_ w358]
          frame False {
          }
          frame True {
            n198 = disable-structure shown="Disabled" {
              disable-tunnel: w358 -> [w359 _]
              frame Disabled {
                n199 = property class="Ctl"(reference=w359, "DisabledEnum"=T7."Disabled and Grayed Out" ("Disabled")) -> ()  [unwired: 1 in, 2 out]
              }
              frame Enabled {
              }
            }
          }
        }
      }
      event User Event {
        n200 = event-data() -> ("CtlRef"=w370:refnum<vi>, "Sub Panel"=w373:refnum<vi>, "This VI"=w372:refnum<vi>, "label"=w369:string)  [unwired: 1 in, 3 out]
        n201 = Match Pattern(string=w369, regular expression=">>" ("search string")) -> (before substring=w367:string, after substring=w366:string)  [unwired: 1 in, 2 out]
        n202 = Equal?(x=w367, y="vi closed" ("label")) -> (x = y?=w364:bool)
        n203 = Equal?(x=w366, y="new vi") -> (x = y?=w363:bool)
        n204 = Not(x=w363) -> (.not. x?=w362:bool)
        n205 = And(x=w364, y=w362) -> (x .and. y?=w361:bool)
        n206 = case shown="True" w364 {
          tunnel: w370 -> [_ w374]
          frame False {
          }
          frame True {
            n207 = property class="Bool (strict)"(reference=w374, "Value"=FALSE) -> (error out=w376:errorcluster)  [unwired: 1 in, 1 out]
            n208 = call <vilib>:"Clear Errors.vi"("error in (no error)"=w376) -> ()  [unwired: 5 in, 2 out]
          }
        }
        n209 = case shown="True" w361 {
          tunnel: w373 -> [_ w383]
          tunnel: w372 -> [_ w382]
          frame False {
          }
          frame True {
            w378 = FALSE ("Visible")
            n210 = invoke class="SubPnl" method="Remove VI"(reference=w383) -> (reference out=w381:refnum<vi>, error out=w379:errorcluster)  [unwired: 2 in, 1 out]
            n211 = disable-structure shown="Enabled" {
              disable-tunnel: w382 -> [w386 _]
              disable-tunnel: [w385 w387] -> w380
              disable-tunnel: w379 -> [w384 w387]
              frame Disabled {
                n212 = Close Reference(reference=w386, error in (no error)=w384) -> (error out=w385:errorcluster)
              }
              frame Enabled {
              }
            }
            n213 = property class="SubPnl"(reference=w381, error in=w380, "Visible"=w378, "Label.Visible"=w378) -> (error out=w377:errorcluster)  [unwired: 1 out]
            n214 = call <vilib>:"Clear Errors.vi"("error in (no error)"=w377) -> ()  [unwired: 5 in, 2 out]
          }
        }
      }
      event "stop": Value Change {
        n215 = event-data() -> ("CtlRef"=w397:refnum<vi>)  [unwired: 1 in, 4 out]
        n216 = Release Queue(queue=w388) -> (error out=w389:errorcluster)  [unwired: 2 in, 2 out]
        n217 = call <vilib>:"Clear Errors.vi"("error in (no error)"=w389) -> ()  [unwired: 5 in, 2 out]
        n218 = property on="DeviceControl" class="Bool (strict)"("Val(Sgnl)"=TRUE ("Value (Signaling)")) -> (error out=w390:errorcluster)  [unwired: 2 in, 1 out]
        n219 = property class="Bool (strict)"(reference=w397, error in=w390, "Value"=FALSE) -> ()  [unwired: 2 out]
        n220 = Generate User Event(user event=w395, event data cluster=T6 {"label"="stop", "Sub Panel"=refnum, "CtlRef"=refnum, "This VI"=refnum} ("event data")) -> (error out=w393:errorcluster)  [unwired: 2 in, 1 out]
        n221 = call <userlib>:"Wait (ms)__ogtk.vi"("error in (no error)"=w393, "milliseconds to wait"=u32 1000) -> ()  [unwired: 8 in, 2 out]
      }
    }
  }
  "Boolean" <- w29
  n222 = while {
    shift-right: [w411] -> _
    shift-left: w31 -> [w405]
    tunnel: w27 -> [_]
    shift-right: ["Position.Channel 7::1"] -> _
    shift-left: _ -> [w402]
    stop <- w407 stop-if-true
    n223 = call "readPlungerStatus.vi"() -> ("read switches"=w412:T1[], "timed out"=w406:bool)  [unwired: 9 in, 1 out]
    n224 = Wait (ms)(milliseconds to wait=u32 100) -> ()  [unwired: 1 out]
    n225 = Not Equal?(x=w405, y=w412) -> (x != y?=w413:bool[])
    n226 = Not Equal?(x="Position.Channel 7::1", y=w402) -> (x != y?=w401:bool)
    n227 = Not(x=w406) -> ()  [unwired: 1 out]
    n228 = Or Array Elements(Boolean array=w413) -> (logical OR=w400:bool)
    n229 = Or(x=w401, y=w400) -> (x .or. y?=w399:bool)
    n230 = case shown="\"Unknown\", Default" "Position.Channel 7::1" {
      tunnel: [plungerstatus."OUT of Beam" ("y") plungerstatus."unknown" ("y") plungerstatus."IN Beam" ("y")] -> w404
      frame "Removed" {
      }
      frame "Unknown", Default {
      }
      frame "Inserted" {
      }
    }
    n231 = case shown="True" w399 {
      tunnel: w412 -> [_ w423]
      tunnel: [w417 w423] -> w411
      tunnel: w405 -> [w417 _]
      tunnel: w404 -> [_ w422]
      frame False {
      }
      frame True {
        n232 = Index Array(array=w423) -> (element #1=→"element":T1, element #2=w436:T1, element #3=w420:T1, element #4=w424:T1)  [unwired: 4 in]
        "Beam Dump 2>>Plunger" <- w436
        "Wedge>>Plunger" <- w420
        "Phosphor>>Plunger" <- w424
        n233 = Equal?(x=w436, y=plungerstatus."IN Beam") -> (x = y?=w421:bool)
        "Beam2" <- w421
        n234 = Equal?(x=w420, y=plungerstatus."OUT of Beam") -> (x = y?=w429:bool)
        n235 = Equal?(x=w424, y=plungerstatus."IN Beam") -> (x = y?=w427:bool)
        n236 = Equal?(x=w422, y=plungerstatus."IN Beam") -> (x = y?=w418:bool)
        "Beam1" <- w418
        n237 = Not(x=w418) -> (.not. x?=w434:bool)
        n238 = Not(x=w421) -> (.not. x?=w433:bool)
        n239 = Or(x=w434, y=w433) -> (x .or. y?=w432:bool)
        n240 = And(x=w432, y=w429) -> (x .and. y?=w426:bool)
        "after Wedge" <- w426
        n241 = Not(x=w426) -> (.not. x?=→"Tele":bool)
        n242 = And(x=w429, y=w427) -> (x .and. y?=→"after Phos":bool)
        "Beam Dump 1>>Plunger" <- w422
      }
    }
    n243 = local read "Boolean"() -> (w408:bool)
    n244 = property on="stop" class="Bool (strict)"() -> ("Value"=w409:bool)  [unwired: 2 in, 2 out]
    n245 = Or(x=w409, y=w408) -> (x .or. y?=w407:bool)
  }
  n246 = Unregister For Events(event registration refnum=w41) -> ()  [unwired: 1 in, 1 out]
  n247 = Destroy User Event(user event=w87) -> ()  [unwired: 1 in, 1 out]
  n248 = DataSocket Close(11:w25) -> ()  [unwired: 2 in, 2 out]
  n249 = for {
    tunnel: w77 -> [w438] mode=indexing
    n250 = Close Reference(reference=w438) -> ()  [unwired: 1 in, 1 out]
  }
  n251 = local write "Boolean"(FALSE ("Boolean")) -> ()
  n252 = Close Reference(reference=w56) -> (error out=w55:errorcluster)  [unwired: 1 in]
  n253 = call <vilib>:"Clear Errors.vi"("error in (no error)"=w55) -> ()  [unwired: 5 in, 2 out]
  "GUIdevice 1" <- "Staging1Wire" ("GUIdevice 12")
  "GUIdevice 2" <- "StagingFocusPositionBeam1" ("GUIdevice 12")
  "GUIdevice 3" <- "StagingFocusPositionBeam2" ("GUIdevice 12")
  "GUIdevice 4" <- "StagingImageLocation" ("GUIdevice 4")
  "GUIdevice 5" <- "StagingShotControl" ("GUIdevice 12")
  "GUIdevice 6" <- "StagingInterlock" ("GUIdevice 12")
  "GUIdevice 7" <- "StagingDelayStage" ("GUIdevice 7")
  "GUIdevice 8" <- "StagingTelescopePosition" ("GUIdevice 12")
  "GUIdevice 9" <- "StagingTRA3" ("GUIdevice 12")
  "GUIdevice 10" <- "StagingBeam1OAPMotors" ("GUIdevice 4")
  "GUIdevice 11" <- "StagingTelescopePosition" ("GUIdevice 4")
  "GUIdevice 12" <- "Staging_USB6210_1" ("GUIdevice 4")
  "GUIdevice 13" <- "SMChydraTT" ("GUIdevice 4")
